vi "NS_NoneModifing.vi"(8 "Error In":errorcluster, 11 "object in":refnum<class "NativeSubTemplate_4x4x4.lvclass">) -> (0 "Error Out":errorcluster, 3 "object out":refnum<class "NativeSubTemplate_4x4x4.lvclass">)   [LabVIEW 2020, in "NativeSubTemplate_4x4x4.lvclass"]
uses:
  NativeSubTemplate_4x4x4.lvclass
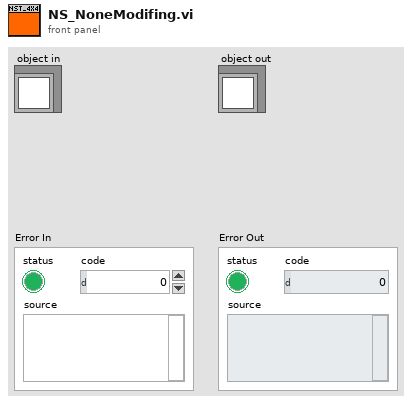
[diagram p1: front panel]
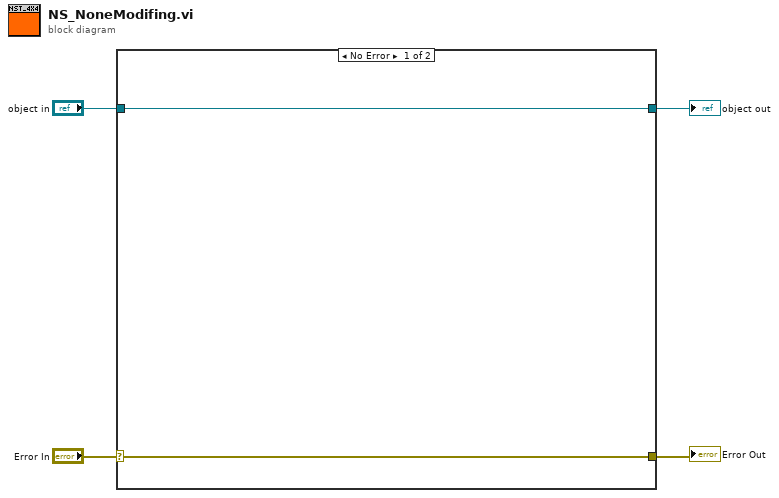
[diagram p0: block diagram]
diagram:
  n1 = case shown="No Error" "Error In" {
    selector: "Error In" -> [w5 w8]
    tunnel: [w5 w8] -> w3
    tunnel: [w6 w7] -> w1
    tunnel: "object in" -> [w6 w7]
    frame No Error {
    }
    frame Error {
    }
  }
  "Error Out" <- w3
  "object out" <- w1
